vi "Set_Pulse_Seq_DAQ.vi"(7 "Time Unit":T1={"Time Unit"=enum."MicroSecond"}, 8 "error in":errorcluster, 9 "Sampling data":T2={"Sample Numbers"=20000000, "Sample  Frequency (Hz)"=20000000}, 10 "Sequence":T3, 11 "Filename (ini)":string="Config_Ver_2\\pulse_sequence_DAQ.ini") -> (0 "error out":errorcluster)   [LabVIEW 2021]
uses:
  DAQ_Control_1.ctl
  DAQ_Control_2.ctl
  DAQ_Control_3 .ctl
  <vilib>/Utility/config.llb/NI_LVConfig.lvlib
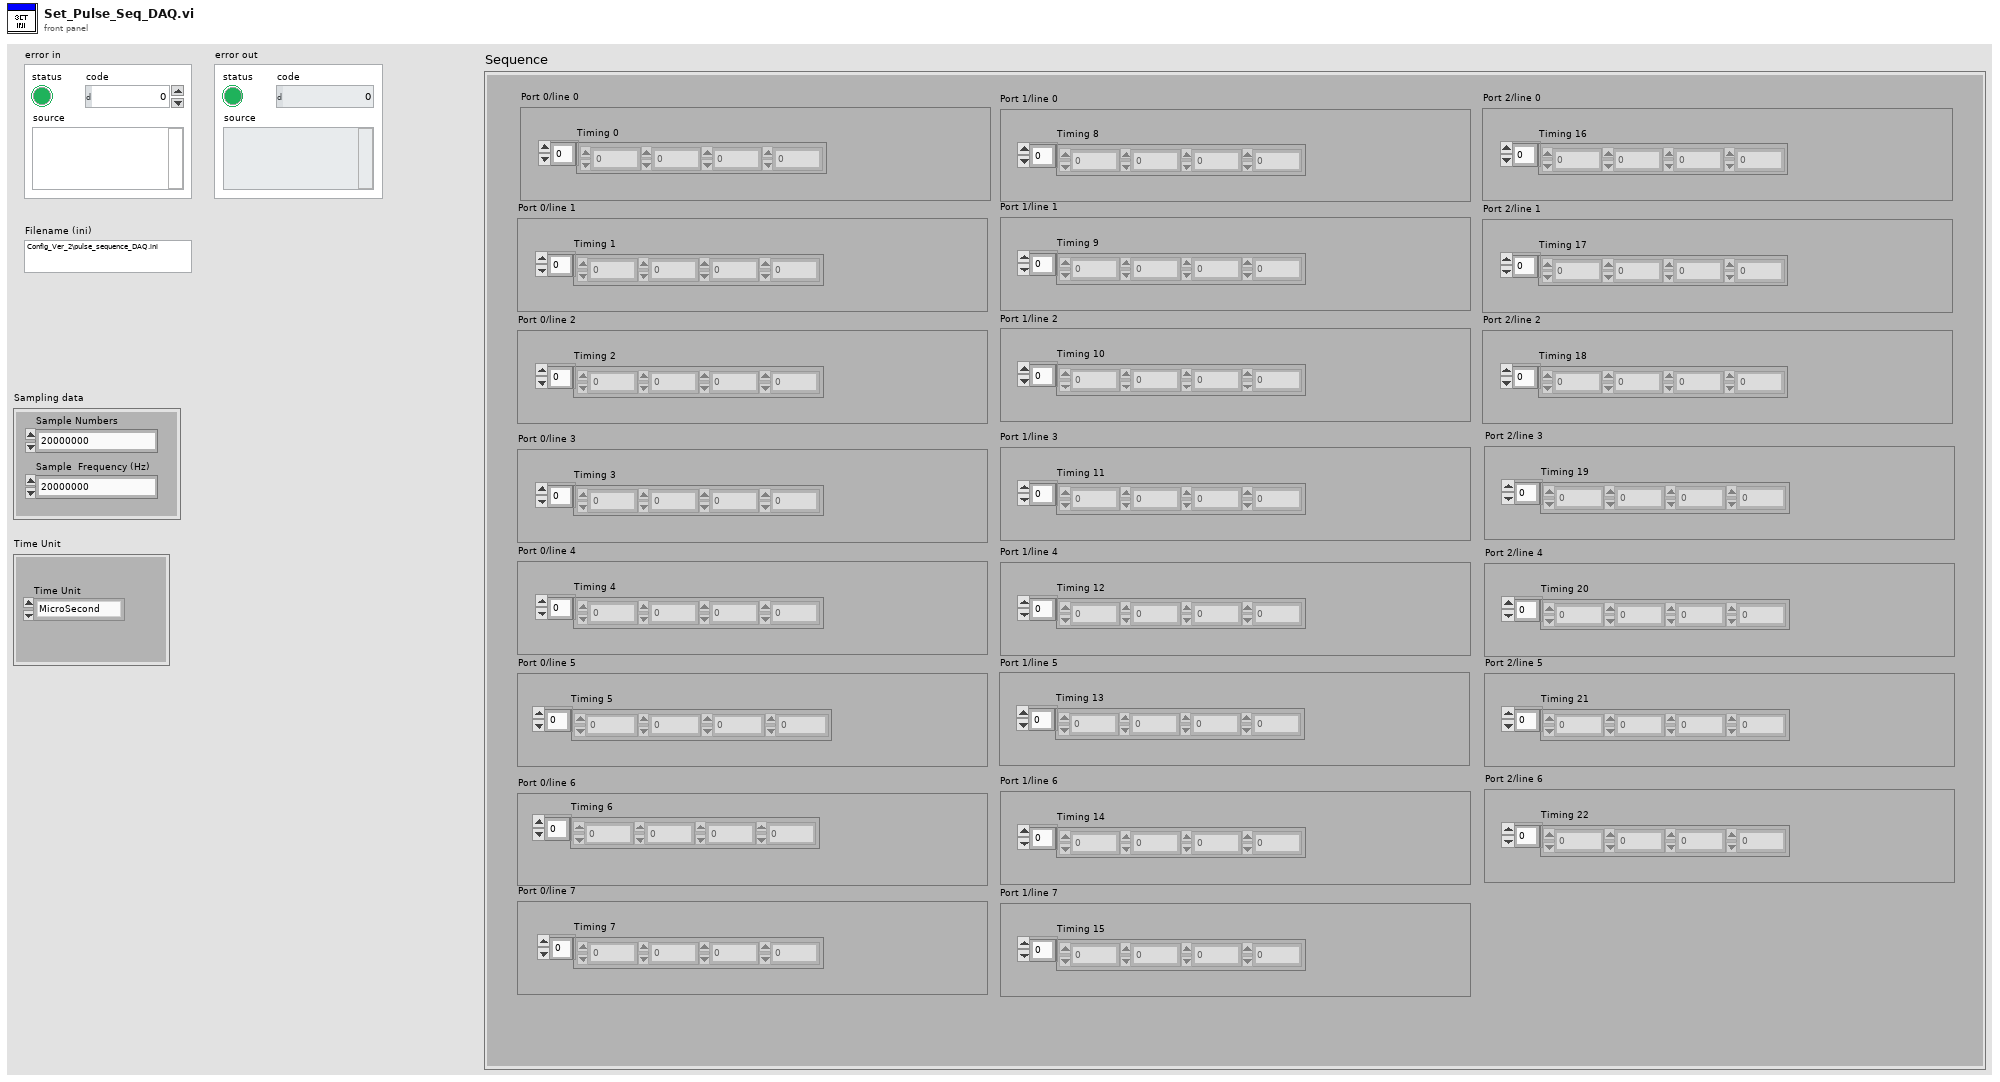
[diagram p1: front panel]
types:
  T1 = typedef "DAQ_Control_3 .ctl" = cluster{"Time Unit":enum16{"NanoSecond", "MicroSecond", "MilliSecond"}}
  T2 = typedef "DAQ_Control_2.ctl" = cluster{"Sample Numbers":u32, "Sample  Frequency (Hz)":u32}
  T3 = typedef "DAQ_Control_1.ctl" = cluster{"Port 2/line 6":cluster{"Timing 22":dbl[]}, "Port 2/line 5":cluster{"Timing 21":dbl[]}, "Port 2/line 4":cluster{"Timing 20":dbl[]}, "Port 2/line 3":cluster{"Timing 19":dbl[]}, "Port 2/line 2":cluster{"Timing 18":dbl[]}, "Port 2/line 1":cluster{"Timing 17":dbl[]}, "Port 2/line 0":cluster{"Timing 16":dbl[]}, "Port 1/line 7":cluster{"Timing 15":dbl[]}, "Port 1/line 6":cluster{"Timing 14":dbl[]}, "Port 1/line 5":cluster{"Timing 13":dbl[]}, "Port 1/line 4":cluster{"Timing 12":dbl[]}, "Port 1/line 3":cluster{"Timing 11":dbl[]}, "Port 1/line 2":cluster{"Timing 10":dbl[]}, "Port 1/line 1":cluster{"Timing 9":dbl[]}, "Port 1/line 0":cluster{"Timing 8":dbl[]}, "Port 0/line 7":cluster{"Timing 7\n":dbl[]}, "Port 0/line 6":cluster{"Timing 6\n":dbl[]}, "Port 0/line 5":cluster{"Timing 5\n":dbl[]}, "Port 0/line 4":cluster{"Timing 4\n":dbl[]}, "Port 0/line 3":cluster{"Timing 3\n":dbl[]}, "Port 0/line 2":cluster{"Timing 2":dbl[]}, "Port 0/line 1":cluster{"Timing 1\n":dbl[]}, "Port 0/line 0":cluster{"Timing 0":dbl[]}}
  T4 = typedef "NI_LVConfig.lvlib/Config Data RefNum.ctl" = refnum<k1>
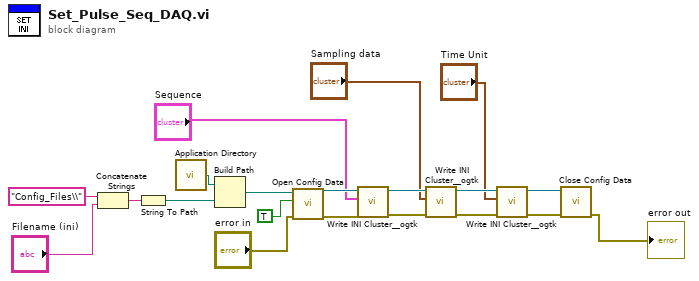
[diagram p0: block diagram]
diagram:
  n1 = Concatenate Strings("Config_Files\\" ("string"), "Filename (ini)") -> (w16:string)
  n2 = String To Path(string=w16) -> (path=w18:path)
  n3 = call <vilib>:"Application Directory.vi"() -> ("Application Directory"=w20:path)
  n4 = Build Path(base path=w20, name or relative path=w18) -> (appended path=w15:path)
  n5 = call <vilib>:"Open Config Data.vi"("error in (no error)"="error in", "create file if necessary (T)"=TRUE, "configuration file path"=w15) -> ("error out"=w12:errorcluster, "refnum"=w11:T4)  [unwired: 6 in, 1 out]
  n6 = call <userlib>:"Write INI Cluster__ogtk.vi"("error in (no error)"=w12, "INI Fomatted Cluster"="Sequence", "refnum"=w11) -> ("error out"=w7:errorcluster, "dup refnum"=w8:T4)  [unwired: 7 in]
  n7 = call <userlib>:"Write INI Cluster__ogtk.vi"("error in (no error)"=w7, "INI Fomatted Cluster"="Sampling data", "refnum"=w8) -> ("error out"=w4:errorcluster, "dup refnum"=w5:T4)  [unwired: 7 in]
  n8 = call <userlib>:"Write INI Cluster__ogtk.vi"("error in (no error)"=w4, "INI Fomatted Cluster"="Time Unit", "refnum"=w5) -> ("error out"=w2:errorcluster, "dup refnum"=w3:T4)  [unwired: 7 in]
  n9 = call <vilib>:"Close Config Data.vi"("error in (no error)"=w2, "refnum"=w3) -> ("error out"=→"error out":errorcluster)  [unwired: 8 in, 1 out]
